vi "UART Close.vi"(8 "error in (no error)":errorcluster) -> (0 "error out":errorcluster)   [LabVIEW 2013]
uses:
  filter wheel/Libraries/uart_library.dll
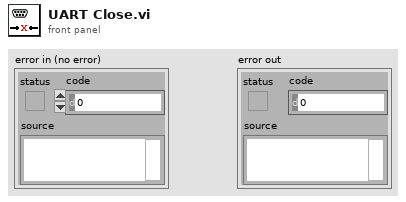
[diagram p1: front panel]
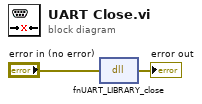
[diagram p0: block diagram]
diagram:
  n1 = dll-call lib="C:/Users/spim/Documents/Labview programs/2014_05_28 SPIM controller mathscript two colour/filter wheel/Libraries/uart_library.dll" fn="fnUART_LIBRARY_close"(error in="error in (no error)") -> (error out=→"error out":errorcluster)  [unwired: 3 in, 1 out]
